vi "optimization2.vi"() -> ()   [LabVIEW 2020]
uses:
  <vilib>/gmath/GlobalOptimization.llb/DE_Settings.ctl
  <vilib>/gmath/GlobalOptimization.llb/DE_Bound Mapping Method.ctl
  <vilib>/gmath/GlobalOptimization.llb/DE_Mutation Method.ctl
  <vilib>/gmath/GlobalOptimization.llb/DE_Crossover Method.ctl
  <vilib>/gmath/GlobalOptimization.llb/DE_Stopping Criteria.ctl
  <vilib>/gmath/GlobalOptimization.llb/DE_State.ctl
  <vilib>/gmath/GlobalOptimization.llb/DE_Population.ctl
  <vilib>/gmath/NI_AAL_GlobalOptimization.lvlib
panel:
  out "Ending State":T1
  in  "Image acquisition time (ms)":dbl=10000.0
  in  "Flyback time (ms)":dbl=10.0
  in  "Bounds":cluster{"Min":dbl[], "Max":dbl[]}={"Min"=[-0.277, 0.503, -0.0581, -0.0216], "Max"=[-0.237, 0.5830000000000001, -0.038099999999999995, -0.001599999999999999]}
  out "VI Type":T3(ring)
  out "number of function calls":i32
  out "Minimum":dbl[](array[numeric])
  out "F(Minimum)":dbl[](array[numeric])
  in  "stopping criteria":T4={"max iterations"=50, "max function calls"=-1, "max time (sec)"=-1.0}
  in  "DE settings":T5={"population size"=10, "scale factor"=0.9, "crossover probability"=0.95, "bound mapping method"=1, "mutation method"=0, "crossover method"=0} {"crossover method" items=["Uniform", "Exponential"]; "mutation method" items=["Random", "Either Or", "Best", "Target to Best"]; "bound mapping method" items=["None", "Random between Bounds and Values", "Re-Initialize"]}
  # "-0.407 + 0.781t + 8.45E-03t^2 + -5.6E-03t^3 =Vout(t)"
  # "=-0.257 + 0.543*F2 + -0.0481*F2^2 + -0.0116*F2^3"
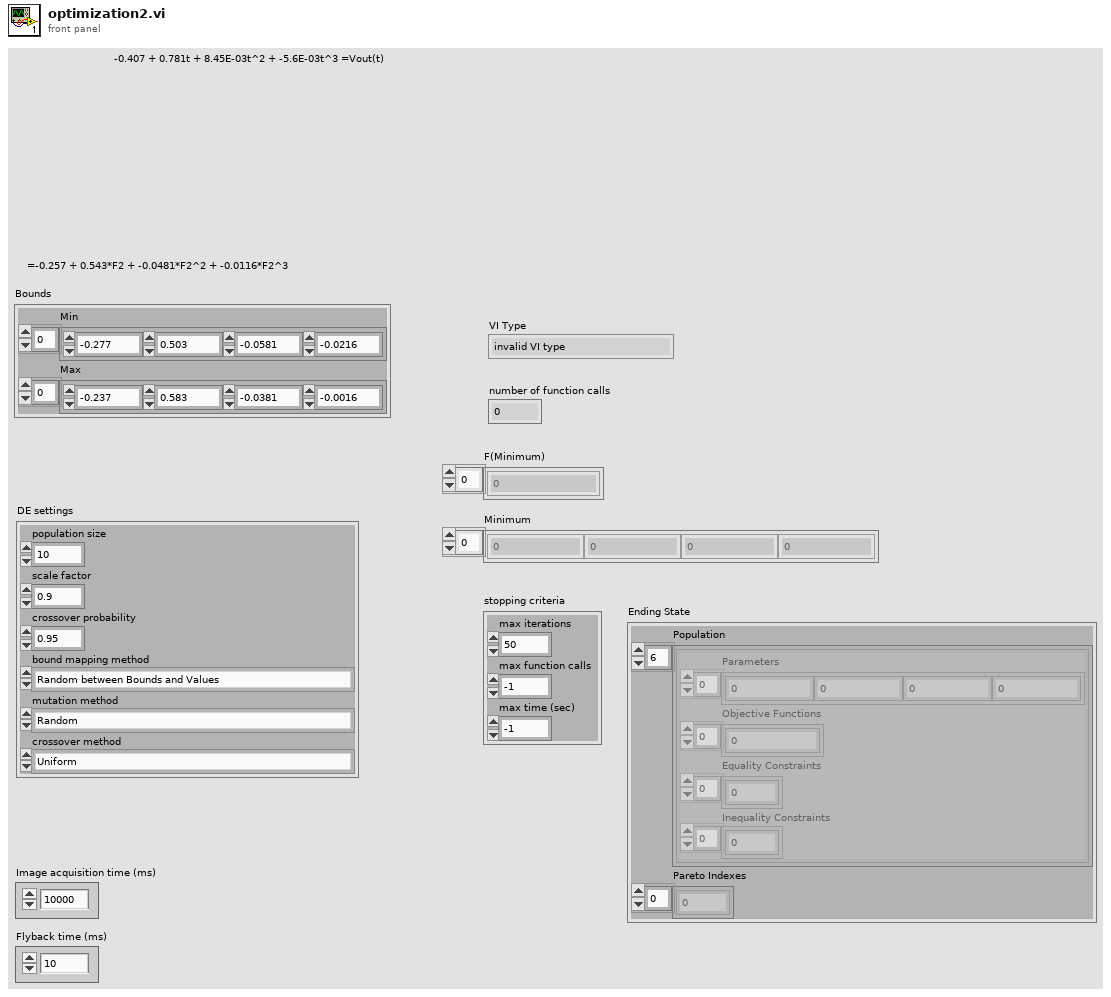
[diagram p1: front panel]
types:
  T1 = typedef "NI_AAL_GlobalOptimization.lvlib/DE_State.ctl" = cluster{"Population":T2[], "Pareto Indexes":i32[]}
  T2 = typedef "NI_AAL_GlobalOptimization.lvlib/DE_Population.ctl" = cluster{"Parameters":dbl[], "Objective Functions":dbl[], "Equality Constraints":dbl[], "Inequality Constraints":dbl[]}
  T3 = enum32{"invalid VI type", "Standard VI", "Control VI", "Global VI", "Polymorphic VI", "Configuration VI", "SubSystem", "Facade VI", "Method VI", "Statechart Diagram VI"}
  T4 = typedef "NI_AAL_GlobalOptimization.lvlib/DE_Stopping Criteria.ctl" = cluster{"max iterations":i32, "max function calls":i32, "max time (sec)":dbl}
  T5 = typedef "NI_AAL_GlobalOptimization.lvlib/DE_Settings.ctl" = cluster{"population size":i32, "scale factor":dbl, "crossover probability":dbl, "bound mapping method":T6, "mutation method":T7, "crossover method":T8}
  T6 = typedef "NI_AAL_GlobalOptimization.lvlib/DE_Bound Mapping Method.ctl" = u16
  T7 = typedef "NI_AAL_GlobalOptimization.lvlib/DE_Mutation Method.ctl" = u16
  T8 = typedef "NI_AAL_GlobalOptimization.lvlib/DE_Crossover Method.ctl" = u16
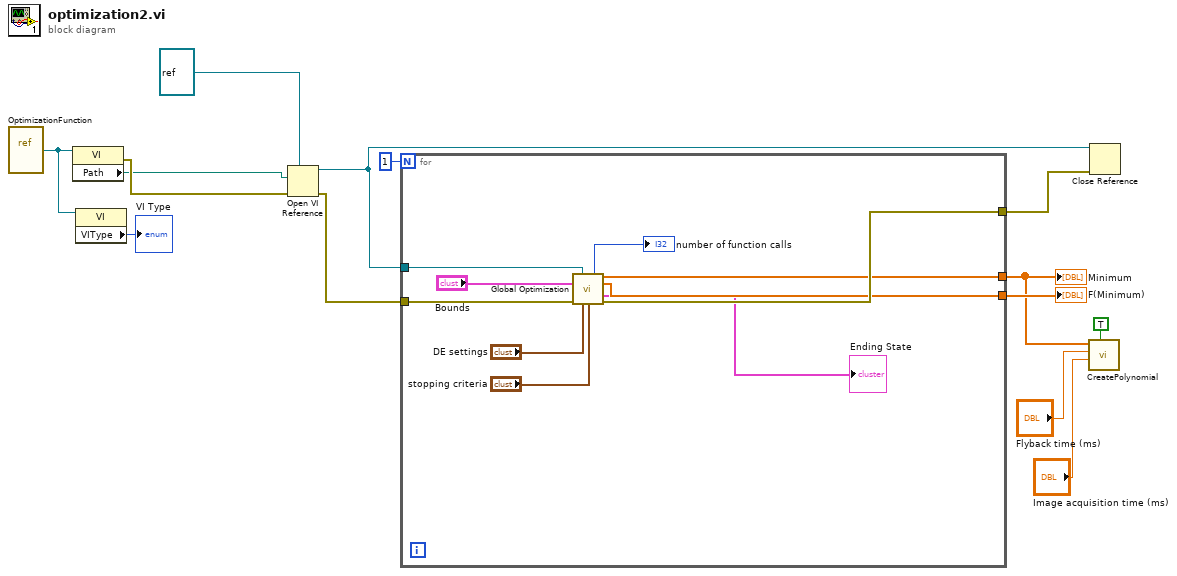
[diagram p0: block diagram]
diagram:
  n1 = vi-ref "OptimizationFunction.vi"() -> (w14:refnum<vi>)
  n2 = property class="VI"(reference=w14) -> (error out=w9:errorcluster, "Path"=w8:path)  [unwired: 1 in, 1 out]
  n3 = property class="VI"(reference=w14) -> ("VIType"=→"VI Type":T3)  [unwired: 1 in, 2 out]
  n4 = Open VI Reference(type specifier VI Refnum (for type only)=refnum<vi> refnum ("objective and constraint function"), vi path=w8, error in (no error)=w9) -> (vi reference=w6:refnum<vi>, error out=w7:errorcluster)  [unwired: 3 in]
  n5 = for {
    N: 1 -> [_]
    tunnel: [w20] -> w11
    tunnel: w7 -> [w19]
    tunnel: w6 -> [w18]
    tunnel: [w17] -> w4
    tunnel: [w16] -> w5
    n6 = call <vilib>:"Global Optimization.vi"("objective and constraint function"=w18, "Bounds"="Bounds", "error in (no error)"=w19, "DE settings"="DE settings", "stopping criteria"="stopping criteria") -> ("number of function calls"=→"number of function calls":i32, "Minimum"=w17:dbl[], "F(Minimum)"=w16:dbl[], "Ending State"=→"Ending State":T1, "error out"=w20:errorcluster)  [unwired: 6 in]
  }
  "F(Minimum)" <- w5
  "Minimum" <- w4
  n7 = call "CreatePolynomial.vi"("Save calibration"=TRUE, "Acquisition time (ms)"="Image acquisition time (ms)", "Flyback (ms)"="Flyback time (ms)", "P(x)"=w4) -> ()  [unwired: 5 in, 2 out]
  n8 = Close Reference(reference=w6, error in (no error)=w11) -> ()  [unwired: 1 out]
